vi "Handle Mouse Down.vi"(4 "PlatMods":T1, 5 "VolatusAPI":refnum<class "VolatusAPI.lvclass">, 6 "Mods":cluster{"Double Click":bool, "Menu Key":bool}, 7 "CtlRef":refnum<vi>, 8 "error in (no error)":errorcluster, 9 "Coords":T2, 10 "Button":u16, 11 "OnMouseDown in":refnum<class "OnMouseDown.lvclass">) -> (0 "error out":errorcluster, 3 "OnMouseDown out":refnum<class "OnMouseDown.lvclass">)   [LabVIEW 2020, in "VolatusGUI.lvlib" / "OnMouseDown.lvclass"]
uses:
  OnMouseDown.lvclass
  <vilib>/Utility/miscctls.llb/LVPoint32TypeDef.ctl
  Volatus/VolatusAPI/VolatusAPI.lvclass
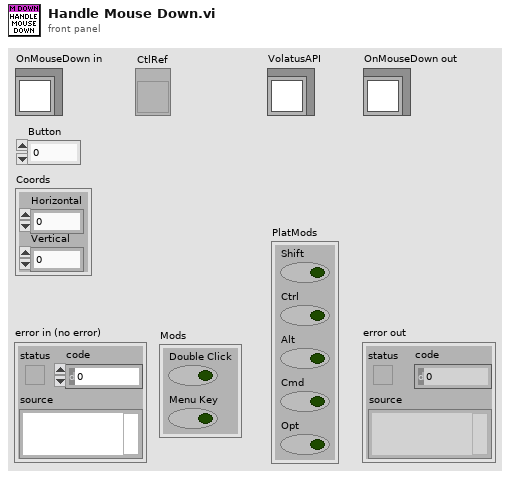
[diagram p1: front panel]
types:
  T1 = cluster{"Shift":bool, "Ctrl":bool, "Alt":bool, "Cmd":bool, "Opt":bool}
  T2 = typedef "LVPoint32TypeDef.ctl" = cluster{"Horizontal":i32, "Vertical":i32}
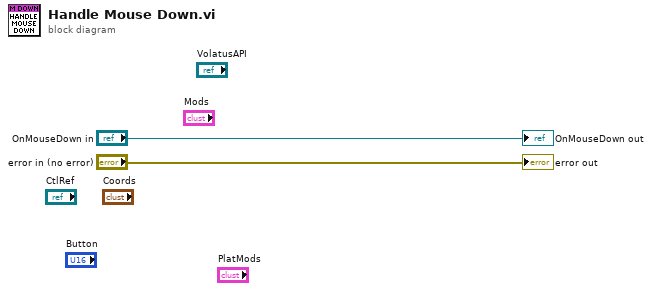
[diagram p0: block diagram]
diagram:
  "error out" <- "error in (no error)"
  "OnMouseDown out" <- "OnMouseDown in"
